vi "PH_Sequencer_Watch.constructor.vi"(0 "name":string, 2 "data in":string, 5 "error in(no error)":errorcluster) -> (14 "i ref out":refnum<vi>, 16 "data out":string, 19 "error out":errorcluster)   [LabVIEW 2014, in "PH_Sequencer_Watch.lvlib"]
doc: "The Sequencer controlles the PHELIX shot procedure.\n\nThis class is part of the PHELIX user layer.\n\nauthor: Stefan Götte, GSI\n\nLicense Agreement for this software:\n\nCopyright (C)\nGesellschaft für Schwerionenforschung, GSI\nPlanckstr. 1\n64291 Darmstadt\nGermany\n\nContact: D.Beck@gsi.de \n\nThis program is free software; you can redistribute it and/or modify it under the terms of the \nGNU General Public License as published by the Free Software Foundation; either version 2 of \nthe license, or (at your option) any later version.\n\nThis program is distributed in the hope that it will be useful, but WITHOUT ANY WARRANTY; \nwithout even the implied warranty of MERCHANTABILITY or FITNESS FOR A PARTICULAR PURPOSE. See the GNU General License for more details (http://www.gnu.org).\n\nGesellschaft für Schwerionenforschung, GSI\nPlanckstr. 1, 64291 Darmstadt, Germany\nFor all questions and ideas contact: M.Richter@gsi.de, H.Brand@gsi.de or D.Beck@gsi.de.\nLast update: 16-JUN-2004"
uses:
  PH_Sequencer_Watch.lvlib
  CS_Core/CSSystem/CSSystemLib/CSSystemLib.lvlib
  CS_Core/CSObj/CSObj.lvlib
  PH_BeamlineInformation/PH_BeamlineInformation.lvlib
  PH_Basics/PH_Common/PH_Common.lvlib
  PH_Basics/PH_Class/PH_Class.lvlib
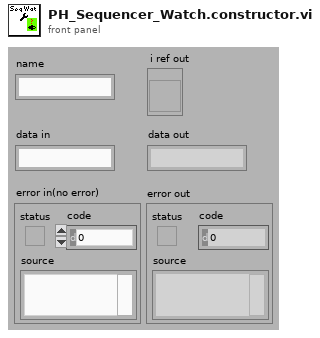
[diagram p1: front panel]
types:
  T1 = enum16{"SetAttribute", "GetAttribute", "CreateAttribute", "DestroyAttribute", "DestroyAllAtributes"}
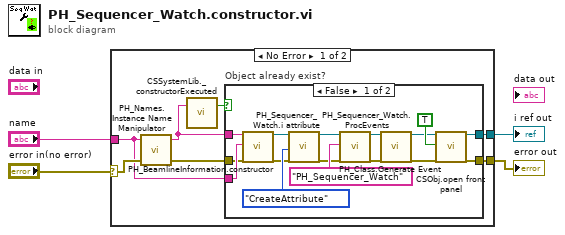
[diagram p0: block diagram]
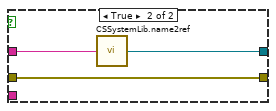
[diagram p2: hidden frame]
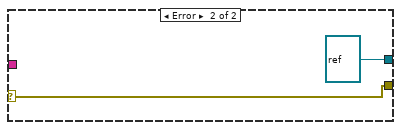
[diagram p3: hidden frame]
diagram:
  n1 = case shown="No Error" "error in(no error)" {
    selector: "error in(no error)" -> [w8 w32]
    tunnel: "name" -> [w5 _]
    tunnel: [w10 w32] -> w3
    tunnel: [w11 refnum<vi> refnum ("i ref out")] -> w2
    frame No Error {
      n2 = call "PH_Names.Instance Name Manipulator.vi"("error in (no error)"=w8, "name in"=w5) -> ("error out"=w7:errorcluster, "name out"=w6:string)  [unwired: 1 in, 1 out]
      n3 = call "CSSystemLib._constructorExecuted.vi"("name"=w6) -> ("constructor executed?"=w9:bool)  [unwired: 18 in]
      n4 = case "Object already exist?" shown="False" w9 {
        tunnel: [w26 w29] -> w11
        tunnel: [w25 w28] -> w10
        tunnel: w6 -> [w27 w30]
        tunnel: w7 -> [w12 w28]
        tunnel: w5 -> [w13 _]
        frame False {
          n5 = call "PH_BeamlineInformation.constructor.vi"("name"=w27, "data in"=w13, "error in(no error)"=w12) -> ("i ref out"=w22:refnum<vi>, "error out"=w21:errorcluster)  [unwired: 14 in, 1 out]
          n6 = call "PH_Sequencer_Watch.i attribute.vi"("VI Refnum"=w22, "Action"=T1."CreateAttribute", "error in (no error)"=w21) -> ("VI Refnum out"=w17:refnum<vi>, "error out"=w15:errorcluster)  [unwired: 14 in, 1 out]
          n7 = call "PH_Class.Generate Event.vi"("i ref in"=w17, "Class"="PH_Sequencer_Watch", "error in (no error)"=w15) -> ("i ref out"=w16:refnum<vi>, "error out"=w14:errorcluster)  [unwired: 15 in]
          n8 = call "PH_Sequencer_Watch.ProcEvents.vi"("i ref in"=w16, "error in (no error)"=w14) -> ("i ref out"=w18:refnum<vi>, "error out"=w19:errorcluster)  [unwired: 16 in]
          n9 = call "CSObj.open front panel.vi"("i ref in"=w18, "frontPanelOpen"=TRUE ("front panel open"), "error in (no error)"=w19) -> ("i ref out"=w26:refnum<vi>, "error out"=w25:errorcluster)  [unwired: 15 in]
        }
        frame True {
          n10 = call "CSSystemLib.name2ref.vi"("name"=w30) -> ("obj refnum"=w29:refnum<vi>)
        }
      }
    }
    frame Error {
    }
  }
  "i ref out" <- w2
  "error out" <- w3
